vi "Panel Size.vi"() -> (0 "Width In Pixels":i32=1200, 3 "Height In pixels":i32=800)   [LabVIEW 2014]
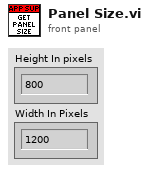
[diagram p1: front panel]
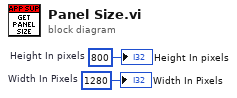
[diagram p0: block diagram]
diagram:
  w1 = 1280  # Width In Pixels
  w2 = 800  # Height In pixels
  "Height In pixels" <- w2
  "Width In Pixels" <- w1
